vi "readFromXML.vi"(8 "error in (no error)":errorcluster, 10 "XML in":string="<MccAzElMove>\n  <azimuth>0.12</azimuth>\n  <elevation>1.5</elevation>\n</MccAzElMove>", 11 "MccAzElMove in":refnum<class "MccAzElMove.lvclass">) -> (0 "error out":errorcluster, 3 "MccAzElMove out":refnum<class "MccAzElMove.lvclass">)   [LabVIEW 2014, in "TCSDataDefinitions.lvlib" / "TCSMountControlCommand.lvlib" / "CommandsForAzElAxes.lvlib" / "MccAzElMove.lvclass"]
uses:
  MccAzElMove.lvclass
  <userlib>/Common/UnitsAndXML/FlattenItemWithUnitToXML/FlattenPlaneAngleToXML/PlaneAngleUnit.ctl
  MccAzElMove.lvclass/MccAzElMove.ctl
  CommandsForAzElAxes.lvclass
  <userlib>/Common/UnitsAndXML/UnitsAndXML.lvlib
  <userlib>/Common/XML/XMLParser/XMLParser.lvclass
panel:
  out "elevation":dbl[unit]=0.026179938779914945
  out "azimuth":dbl[unit]=0.0020943951023931952
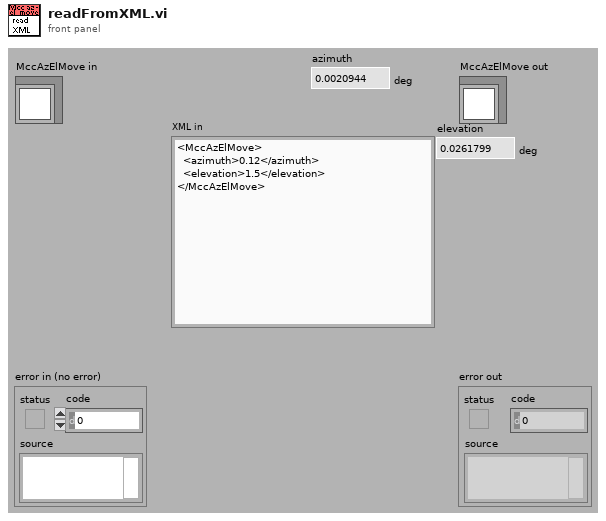
[diagram p1: front panel]
types:
  T1 = typedef "UnitsAndXML.lvlib/PlaneAngleUnit.ctl" = enum16{"rad", "deg", "'", "\""}
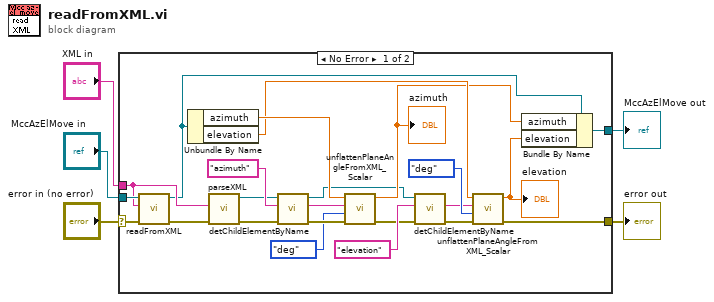
[diagram p0: block diagram]
diagram:
  n1 = case shown="No Error" "error in (no error)" {
    selector: "error in (no error)" -> [w28 w30]
    tunnel: [w8 w30] -> w4
    tunnel: [w20 w29] -> w2
    tunnel: "MccAzElMove in" -> [w27 w29]
    tunnel: "XML in" -> [w26 _]
    frame No Error {
      n2 = call-parent "readFromXML.vi"("error in (no error)"=w28, "XML in"=w26, "CommandsForAzElAxes in"=w27) -> ("error out"=w25:errorcluster, "CommandsForAzElAxes out"=w21:refnum<class "MccAzElMove.lvclass">)  [unwired: 7 out]
      n3 = Unbundle By Name(w21) -> ("azimuth"=w18:dbl[unit], "elevation"=w11:dbl[unit])
      n4 = call <userlib>:"parseXML.vi"("error in (no error)"=w25, "XMLString in"=w26) -> ("error out"=w24:errorcluster, "Element out"=w7:refnum<class "XMLParser.lvclass">)  [unwired: 8 in]
      n5 = call <userlib>:"detChildElementByName.vi"("error in (no error)"=w24, "childName"="azimuth" ("ChildName"), "Element in"=w7) -> ("error out"=w17:errorcluster, "childXML"=w19:string, "Element out"=w6:refnum<class "XMLParser.lvclass">)  [unwired: 5 in, 1 out]
      n6 = call <userlib>:"unflattenPlaneAngleFromXML_Scalar.vi"("error in (no error)"=w17, "planeAngleUnitInXML"=PlaneAngleUnit."deg", "xmlString"=w19, "planeAngleForType"=w18) -> ("error out"=w16:errorcluster, "planeAngle"=w10:dbl[unit])  [unwired: 6 in]
      "azimuth" <- w10
      n7 = call <userlib>:"detChildElementByName.vi"("error in (no error)"=w16, "childName"="elevation" ("ChildName"), "Element in"=w6) -> ("error out"=w12:errorcluster, "childXML"=w13:string)  [unwired: 5 in, 2 out]
      n8 = call <userlib>:"unflattenPlaneAngleFromXML_Scalar.vi"("error in (no error)"=w12, "planeAngleUnitInXML"=PlaneAngleUnit."deg", "xmlString"=w13, "planeAngleForType"=w11) -> ("error out"=w8:errorcluster, "planeAngle"=w9:dbl[unit])  [unwired: 6 in]
      "elevation" <- w9
      n9 = Bundle By Name(cluster=w21, "azimuth"=w10, "elevation"=w9) -> (w20:refnum<class "MccAzElMove.lvclass">)
    }
    frame Error {
    }
  }
  "error out" <- w4
  "MccAzElMove out" <- w2
